vi "Divide XY (single).vi"(8 "error in (no error)":errorcluster, 9 "y":cluster{"X-array":dbl[], "Y-array":dbl[]}, 11 "XY-data":cluster{"X-array":dbl[], "Y-array":dbl[]}) -> (0 "error out":errorcluster, 3 "XY-data out":cluster{"X-array":dbl[], "Y-array":dbl[]} {"Y-array" format="%.2p"; "X-array" format="%.2p"})   [LabVIEW 2019, in "xy_utilities.lvlib"]
doc: "Divide <b>y</b>'s y array by the y array of <b>XY-data</b>.\n\nWire data to the data input to determine the polymorphic instance to use or manually select the instance."
uses:
  xy_utilities.lvlib
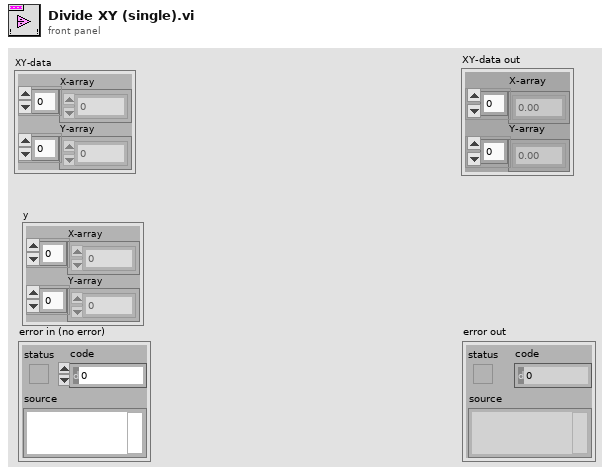
[diagram p1: front panel]
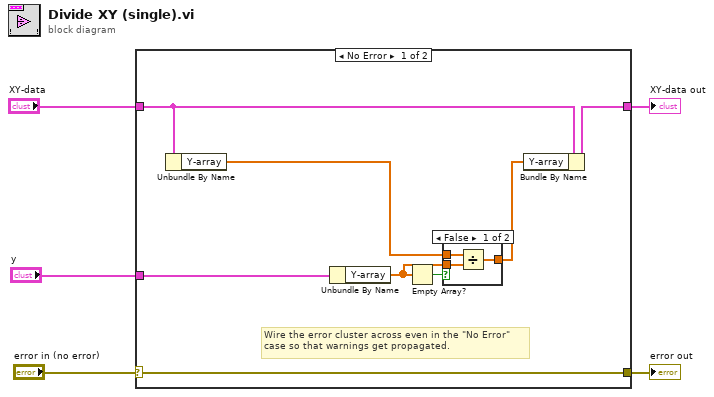
[diagram p0: block diagram]
diagram:
  n1 = case shown="No Error" "error in (no error)" {
    selector: "error in (no error)" -> [w13 w19]
    tunnel: [w13 w19] -> w4
    tunnel: "XY-data" -> [w12 w18]
    tunnel: [w11 w18] -> w2
    tunnel: "y" -> [w10 _]
    frame No Error {
      # "Wire the error cluster across even in the \"No Error\"\ncase so that warnings get propagated."
      n2 = Unbundle By Name(w12) -> ("Y-array"=w7:dbl[])
      n3 = Unbundle By Name(w10) -> ("Y-array"=w8:dbl[])
      n4 = Empty Array?(array=w8) -> (empty?=w9:bool)
      n5 = case shown="False" w9 {
        tunnel: w8 -> [w16 _]
        tunnel: w7 -> [w15 w17]
        tunnel: [w14 w17] -> w6
        frame False {
          n6 = Divide(x=w15, y=w16) -> (x/y=w14:dbl[])
        }
        frame True {
        }
      }
      n7 = Bundle By Name(cluster=w12, "Y-array"=w6) -> (w11:cluster{"X-array":dbl[], "Y-array":dbl[]})
    }
    frame Error {
    }
  }
  "error out" <- w4
  "XY-data out" <- w2
